vi "Config Default.vi"() -> (0 "System Config Out":T1={"System Ver"=0, "Auto Angle PID"={"Gains"={"P"=0.1, "I"=0.0, "D"=0.0, "F"=0.0}, "Error Allowed"={"High"=2.0, "Low"=-2.0}, "I Zone"={"High"=0.0, "Low"=0.0}, "Peak Out 0-1"={"High"=1.0, "Low"=-1.0}, "Max I Accu"={"High"=0.0, "Low"=0.0}}, "Frame"={"Length"=33.0, "Width"=18.0}, "Drive Data"={"CPR"=14.0, "RevMotor/Wheel"=6.67, "Wheel Diameter (in)"=4.0}, "Speed Full Scale"=5000.0, "Steer Data"={"CPR"=1024.0}} {"Auto Angle PID"."Max I Accu"."Low" format="%#.8f"; "Auto Angle PID"."Max I Accu"."High" format="%#.8f"; "Auto Angle PID"."Gains"."F" format="%#.8f"; "Auto Angle PID"."Gains"."D" format="%#.8f"; "Auto Angle PID"."Gains"."I" format="%#.8f"; "Auto Angle PID"."Gains"."P" format="%#.8f"; "Auto Angle PID"."Error Allowed"."Low" format="%#.8f"; "Auto Angle PID"."Error Allowed"."High" format="%#.8f"; "Auto Angle PID"."I Zone"."Low" format="%#.8f"; "Auto Angle PID"."I Zone"."High" format="%#.8f"; "Auto Angle PID"."Peak Out 0-1"."Low" format="%#.8f"; "Auto Angle PID"."Peak Out 0-1"."High" format="%#.8f"}, 1 "Drive Default Out":T11={"Drive HW Ver"=0, "SparkMax Output"={"Motor Invert"=FALSE, "Ramp Rate OL (S)"=1.0, "Dead Band"=0.0, "Idle Mode"=enum."Coast"}, "Slot 0 CL"={"Gains"={"P"=0.1, "I"=0.0, "D"=0.0, "F"=0.0}, "I Zone"=0.0, "Peak Out -1 0 1"={"High"=1.0, "Low"=-1.0}, "Max I Accu"=0.0}, "Slot 0 SM"={"Max Velocity"=2000.0, "Max Acceleration"=5000.0, "Allowed CL Error"=0.0, "Min Velocity Output"=0.0}} {"Slot 0 CL"."Gains"."F" format="%#.8f"; "Slot 0 CL"."Gains"."D" format="%#.8f"; "Slot 0 CL"."Gains"."I" format="%#.8f"; "Slot 0 CL"."Gains"."P" format="%#.8f"; "Slot 0 CL"."Peak Out -1 0 1"."Low" format="%#.8f"; "Slot 0 CL"."Peak Out -1 0 1"."High" format="%#.8f"}, 2 "Steer Default Out":T16={"Steer HW Ver"=0, "SRX Output"={"Neutral"=enum."Override to Coast", "Max"={"FWD"=1.0, "REV"=-1.0}, "Min"={"FWD"=0.0, "REV"=0.0}, "OL Ramp Rate (S)"=1.0, "Dead Band"=0.02, "CL Ramp Rate (S)"=1.0}, "Slot 0 CL"={"Gains"={"P"=0.5, "I"=0.0, "D"=0.0, "F"=0.0}, "Error Allowed"=2.0, "I Zone"=0.0, "Peak Out 0-1"=1.0, "Max I Accu"=0.0}, "Slot 0 MM"={"Cruise Velocity"=0, "Acceleration"=0}} {"Slot 0 CL"."Gains"."F" format="%#.8f"; "Slot 0 CL"."Gains"."D" format="%#.8f"; "Slot 0 CL"."Gains"."I" format="%#.8f"; "Slot 0 CL"."Gains"."P" format="%#.8f"; "SRX Output"."Min"."REV" format="%.2f"; "SRX Output"."Min"."FWD" format="%.2f"; "SRX Output"."Max"."REV" format="%.2f"; "SRX Output"."Max"."FWD" format="%.2f"}, 3 "Module Specific Default Out":T8={"Specific HW Ver"=0, "Specific Data"=[{"Motor Pos"=enum."Left-Front", "CAN Bus"="", "Drive ID"=1, "Steer ID"=0, "Encoder Start Value"=1.0}, {"Motor Pos"=enum."Right-Front", "CAN Bus"="", "Drive ID"=2, "Steer ID"=0, "Encoder Start Value"=2.0}, {"Motor Pos"=enum."Right-Back", "CAN Bus"="", "Drive ID"=3, "Steer ID"=0, "Encoder Start Value"=3.0}, {"Motor Pos"=enum."Left-Back", "CAN Bus"="", "Drive ID"=4, "Steer ID"=0, "Encoder Start Value"=4.0}]})   [LabVIEW 2023, in "Swerve-SteerSRX-DriveSpark-AbsAnalog_ACT.lvlib"]
uses:
  Swerve-SteerSRX-DriveSpark-AbsAnalog_ACT.lvlib
  Cluster_Config Steer HW Values.ctl
  Shared Code/TypeDefs/Cluster_Config SRX Motor Output.ctl
  <vilib>/Rock Robotics/WPI/ThirdParty/Phoenix-LabVIEW/Motor Controller/Controls/CTRE_Phoenix_MotorControl_NeutralMode.ctl
  Shared Code/TypeDefs/Cluster_FWD  REV Values.ctl
  Shared Code/TypeDefs/Cluster_SRX SLOT PID Config.ctl
  Shared Code/TypeDefs/Cluster_PID Gains.ctl
  Shared Code/TypeDefs/Cluster_SRX Motion Magic Parameters.ctl
  Cluster_Config Drive HW Values.ctl
  Shared Code/TypeDefs/Cluster_SparkMax Config_Motor Output.ctl
  <vilib>/Rock Robotics/WPI/ThirdParty/REV Robotics/REVLib/Typedef/Spark MAX Idle Mode.ctl
  Shared Code/TypeDefs/Cluster_Spark MAX Config_SLOT PID Config.ctl
  Shared Code/TypeDefs/Cluster_High-Low.ctl
  Shared Code/TypeDefs/Cluster_SparkMax Config_Smart Motion Parameters.ctl
  Cluster_Config Specific HW Values.ctl
  Cluster_Config Specific Data.ctl
  Shared Code/TypeDefs/ENUM_Module Position.ctl
  Cluster_System Config_Values.ctl
  Shared Code/TypeDefs/Cluster_SW PID Config.ctl
  Type Defs/Cluster_Length and Width.ctl
  Shared Code/TypeDefs/Cluster_Config_Swerve_Drive Param.ctl
  Shared Code/TypeDefs/Cluster_Config_Swerve_Steer Parm.ctl
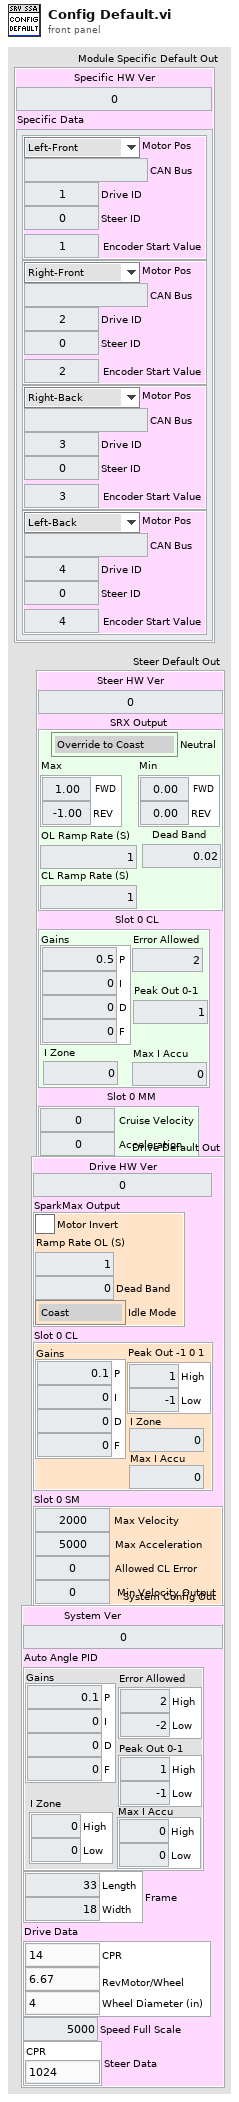
[diagram p1: front panel]
types:
  T1 = typedef "Swerve-SteerSRX-DriveSpark-AbsAnalog_ACT.lvlib/Cluster_System Config_Values.ctl" = cluster{"System Ver":u64, "Auto Angle PID":T2, "Frame":T5, "Drive Data":T6, "Speed Full Scale":dbl, "Steer Data":T7}
  T2 = typedef "Cluster_SW PID Config.ctl" = cluster{"Gains":T3, "Error Allowed":T4, "I Zone":T4, "Peak Out 0-1":T4, "Max I Accu":T4}
  T3 = typedef "Cluster_PID Gains.ctl" = cluster{"P":dbl, "I":dbl, "D":dbl, "F":dbl}
  T4 = typedef "Cluster_High-Low.ctl" = cluster{"High":dbl, "Low":dbl}
  T5 = typedef "Cluster_Length and Width.ctl" = cluster{"Length":dbl, "Width":dbl}
  T6 = typedef "Cluster_Config_Swerve_Drive Param.ctl" = cluster{"CPR":dbl, "RevMotor/Wheel":dbl, "Wheel Diameter (in)":dbl}
  T7 = typedef "Cluster_Config_Swerve_Steer Parm.ctl" = cluster{"CPR":dbl}
  T8 = typedef "Swerve-SteerSRX-DriveSpark-AbsAnalog_ACT.lvlib/Cluster_Config Specific HW Values.ctl" = cluster{"Specific HW Ver":u64, "Specific Data":T9[]}
  T9 = typedef "Swerve-SteerSRX-DriveSpark-AbsAnalog_ACT.lvlib/Cluster_Config Specific Data.ctl" = cluster{"Motor Pos":T10, "CAN Bus":string, "Drive ID":u8, "Steer ID":u8, "Encoder Start Value":dbl}
  T10 = typedef "ENUM_Module Position.ctl" = enum16{"Left-Front", "Right-Front", "Left-Back", "Right-Back"}
  T11 = typedef "Swerve-SteerSRX-DriveSpark-AbsAnalog_ACT.lvlib/Cluster_Config Drive HW Values.ctl" = cluster{"Drive HW Ver":u64, "SparkMax Output":T12, "Slot 0 CL":T14, "Slot 0 SM":T15}
  T12 = typedef "Cluster_SparkMax Config_Motor Output.ctl" = cluster{"Motor Invert":bool, "Ramp Rate OL (S)":dbl, "Dead Band":dbl, "Idle Mode":T13}
  T13 = typedef "Spark MAX Idle Mode.ctl" = enum16{"Coast", "Brake"}
  T14 = typedef "Cluster_Spark MAX Config_SLOT PID Config.ctl" = cluster{"Gains":T3, "I Zone":dbl, "Peak Out -1 0 1":T4, "Max I Accu":dbl}
  T15 = typedef "Cluster_SparkMax Config_Smart Motion Parameters.ctl" = cluster{"Max Velocity":dbl, "Max Acceleration":dbl, "Allowed CL Error":dbl, "Min Velocity Output":dbl}
  T16 = typedef "Swerve-SteerSRX-DriveSpark-AbsAnalog_ACT.lvlib/Cluster_Config Steer HW Values.ctl" = cluster{"Steer HW Ver":u64, "SRX Output":T17, "Slot 0 CL":T20, "Slot 0 MM":T21}
  T17 = typedef "Cluster_Config SRX Motor Output.ctl" = cluster{"Neutral":T18, "Max":T19, "Min":T19, "OL Ramp Rate (S)":dbl, "Dead Band":dbl, "CL Ramp Rate (S)":dbl}
  T18 = typedef "CTRE_Phoenix_MotorControl_NeutralMode.ctl" = enum8{"EEPROMSetting", "Override to Coast", "Override to Brake"}
  T19 = typedef "Cluster_FWD  REV Values.ctl" = cluster{"FWD":dbl, "REV":dbl}
  T20 = typedef "Cluster_SRX SLOT PID Config.ctl" = cluster{"Gains":T3, "Error Allowed":dbl, "I Zone":dbl, "Peak Out 0-1":dbl, "Max I Accu":dbl}
  T21 = typedef "Cluster_SRX Motion Magic Parameters.ctl" = cluster{"Cruise Velocity":i32, "Acceleration":i32}
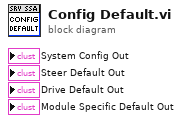
[diagram p0: block diagram]
diagram:
